vi "BRAM_ReadScore.vi"(1 "Player":u8, 4 "Address":i16) -> (16 "PixelData":bool[](array[boolean]))   [LabVIEW 2018]
uses:
  <vilib>/rvi/Memory/Memory_Emulation/nirvimemoryFastEmulation.vi
  <vilib>/rvi/Memory/Memory_Emulation/nirvimemoryEmulation.vi
  <vilib>/rvi/Emulation/niFpgaEmulationIsFPGAContextNoSignature.vi
  <vilib>/rvi/DataTransferAndStorage/Container/Common/niFpgaContainerGetUniqueNameForEmu.vi
  <vilib>/rvi/Emulation/niFpgaProcessEmulError.vi
  <vilib>/rvi/Emulation/niFpgaSctlEmulationGetInTimedLoop.vi
  <vilib>/rvi/errors/nirviReportUnexpectedCaseInternalError (U32).vi
  <vilib>/rvi/DataTransferAndStorage/Container/XNode/niFpgaContainer.xnode
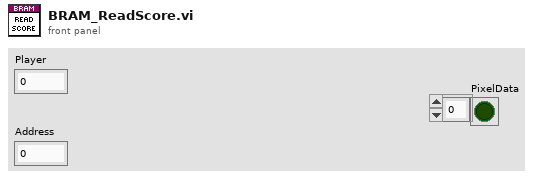
[diagram p1: front panel]
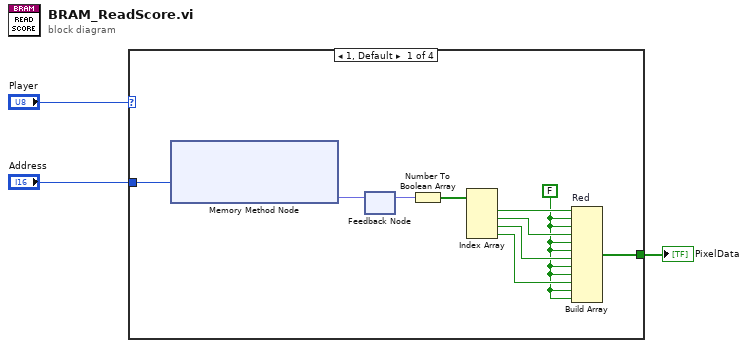
[diagram p0: block diagram]
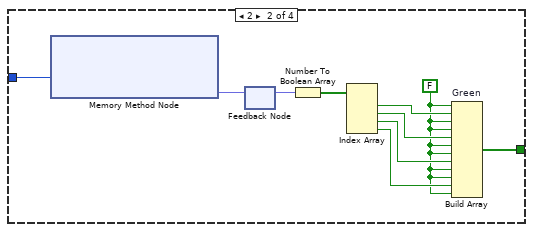
[diagram p2: hidden frame]
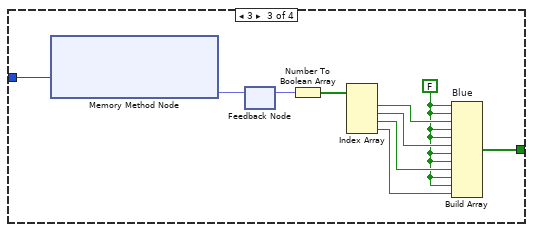
[diagram p3: hidden frame]
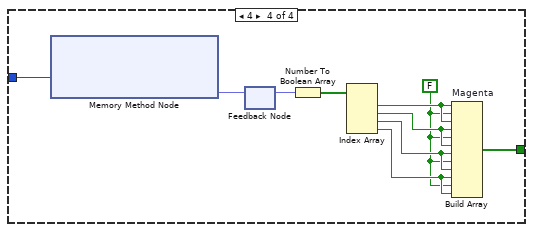
[diagram p4: hidden frame]
diagram:
  n1 = case shown="1, Default" "Player" {
    tunnel: "Address" -> [w13 w23 w33 w43]
    tunnel: [w4 w19 w29 w39] -> w1
    frame 1, Default {
      w5 = FALSE
      n2 = xnode ("Memory Method Node")("Address"=w13) -> ("Data"=w12:fxp<+,4,4>)  [unwired: 1 in, 1 out]
      n3 = feedback #1() -> (w11:fxp<+,4,4>)  [unwired: 1 in]
      n4 = feedback-in #1(w12) -> ()
      n5 = Number To Boolean Array(number=w11) -> (Boolean array=w10:bool[])
      n6 = Index Array(array=w10) -> (element #1=w9:bool, element #2=w8:bool, element #3=w7:bool, element #4=w6:bool)  [unwired: 4 in]
      n7 = Build Array "Red"(w9, w5, w5, w8, w5, w5, w7, w5, w5, w6, w5, w5) -> (w4:bool[])
    }
    frame 2 {
      w14 = FALSE
      n8 = xnode ("Memory Method Node")("Address"=w23) -> ("Data"=w22:fxp<+,4,4>)  [unwired: 1 in, 1 out]
      n9 = feedback #2() -> (w21:fxp<+,4,4>)  [unwired: 1 in]
      n10 = feedback-in #2(w22) -> ()
      n11 = Number To Boolean Array(number=w21) -> (Boolean array=w20:bool[])
      n12 = Index Array(array=w20) -> (element #1=w18:bool, element #2=w17:bool, element #3=w16:bool, element #4=w15:bool)  [unwired: 4 in]
      n13 = Build Array "Green"(w14, w18, w14, w14, w17, w14, w14, w16, w14, w14, w15, w14) -> (w19:bool[])
    }
    frame 3 {
      w24 = FALSE
      n14 = xnode ("Memory Method Node")("Address"=w33) -> ("Data"=w32:fxp<+,4,4>)  [unwired: 1 in, 1 out]
      n15 = feedback #3() -> (w31:fxp<+,4,4>)  [unwired: 1 in]
      n16 = feedback-in #3(w32) -> ()
      n17 = Number To Boolean Array(number=w31) -> (Boolean array=w30:bool[])
      n18 = Index Array(array=w30) -> (element #1=w28:bool, element #2=w27:bool, element #3=w26:bool, element #4=w25:bool)  [unwired: 4 in]
      n19 = Build Array "Blue"(w24, w24, w28, w24, w24, w27, w24, w24, w26, w24, w24, w25) -> (w29:bool[])
    }
    frame 4 {
      w34 = FALSE
      n20 = xnode ("Memory Method Node")("Address"=w43) -> ("Data"=w42:fxp<+,4,4>)  [unwired: 1 in, 1 out]
      n21 = feedback #4() -> (w41:fxp<+,4,4>)  [unwired: 1 in]
      n22 = feedback-in #4(w42) -> ()
      n23 = Number To Boolean Array(number=w41) -> (Boolean array=w40:bool[])
      n24 = Index Array(array=w40) -> (element #1=w38:bool, element #2=w37:bool, element #3=w36:bool, element #4=w35:bool)  [unwired: 4 in]
      n25 = Build Array "Magenta"(w38, w34, w38, w37, w34, w37, w36, w34, w36, w35, w34, w35) -> (w39:bool[])
    }
  }
  "PixelData" <- w1
